vi "Serial Command Test App.vi"() -> ()   [LabVIEW 2011]
uses:
  <vilib>/Instr/_visa.llb/VISA Configure Serial Port (Instr).vi
panel:
  out "concatenated string":string
  in  "Command":string
  in  "Stop Button":bool
  in  "Send":bool
  in  "VISA resource name 2":refnum<visa-resource-name>
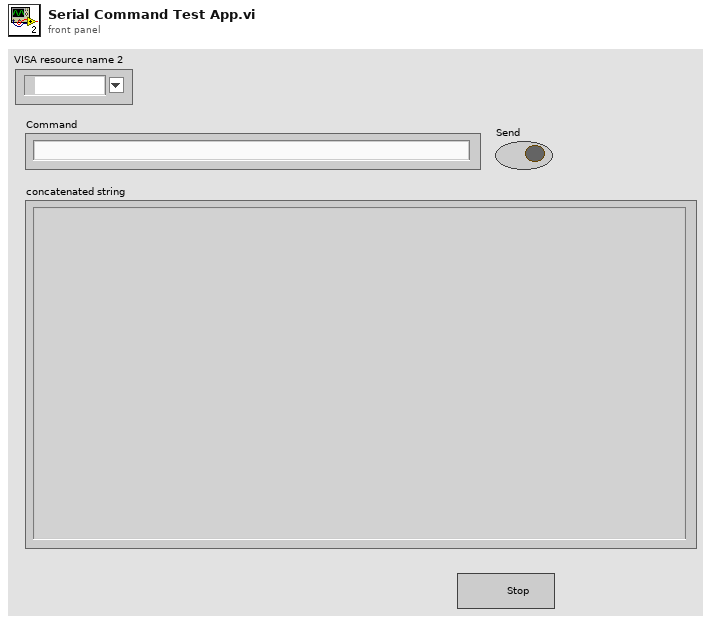
[diagram p1: front panel]
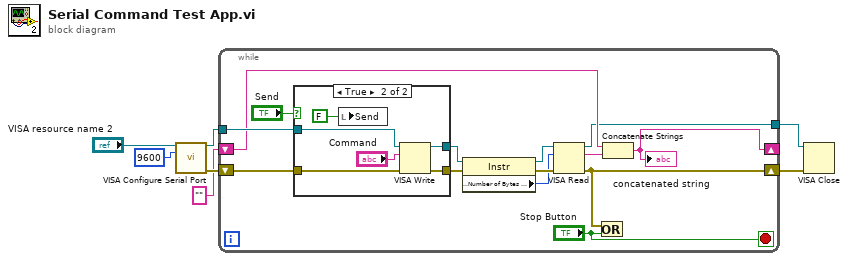
[diagram p0: block diagram]
diagram:
  n1 = call-poly "VISA Configure Serial Port"("VISA resource name"="VISA resource name 2", "baud rate (9600)"=u32 9600) -> ("VISA resource name out"=w7:refnum<visa-resource-name>, "error out"=w4:errorcluster)  [unwired: 12 in]
  n2 = while {
    tunnel: w7 -> [w21]
    shift-right: [w8] -> w1
    shift-left: w4 -> [w20]
    shift-right: [w9] -> _
    shift-left: "" -> [w12]
    tunnel: [w10] -> w2
    stop <- "Stop Button" stop-if-true
    n3 = case shown="True" "Send" {
      tunnel: w21 -> [w23 w29]
      tunnel: w20 -> [w22 w28]
      tunnel: [w23 w24] -> w14
      tunnel: [w22 w26] -> w13
      frame False {
      }
      frame True {
        n4 = local write "Send"(FALSE ("Send")) -> ()
        n5 = VISA Write(VISA resource name=w29, write buffer="Command", error in (no error)=w28) -> (VISA resource name out=w24:refnum<visa-resource-name>, error out=w26:errorcluster)  [unwired: 1 out]
      }
    }
    n6 = property class="Instr"(reference=w14, error in=w13) -> (reference out=w17:refnum<visa-resource-name>, error out=w16:errorcluster, "Serial Settings:Number of Bytes at Serial Port"=w15:u32)
    n7 = VISA Read(VISA resource name=w17, byte count=w15, error in (no error)=w16) -> (VISA resource name out=w10:refnum<visa-resource-name>, read buffer=w11:string, error out=w8:errorcluster)  [unwired: 1 out]
    n8 = Or(x=w8, y="Stop Button") -> ()  [unwired: 1 out]
    n9 = Concatenate Strings(w12, w11) -> (w9:string)
    "concatenated string" <- w9
  }
  n10 = VISA Close(VISA resource name=w2, error in (no error)=w1) -> ()  [unwired: 1 out]
